vi "resampleA.vi"(8 "error in (no error)":errorcluster, 11 "Waveform":waveform(dbl)) -> (0 "error out":errorcluster, 3 "resampled waveform out":waveform(dbl))   [LabVIEW 2018]
uses:
  <vilib>/measure/maresamp.llb/Resample Waveform (single shot).vi
  <vilib>/measure/NI_MAPro.lvlib
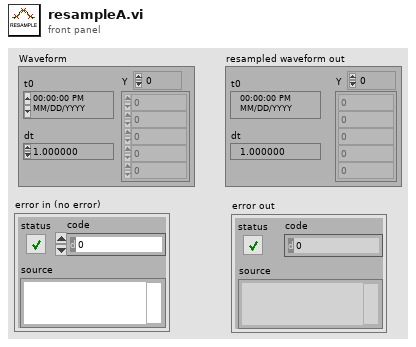
[diagram p1: front panel]
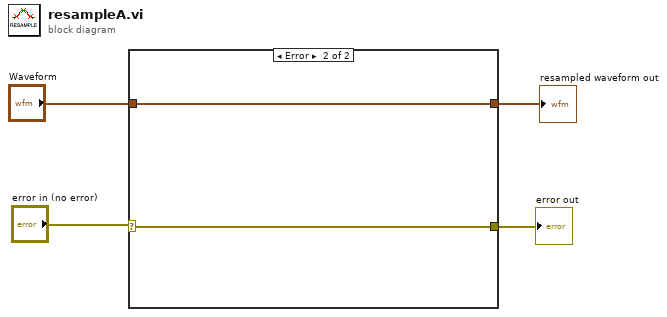
[diagram p0: block diagram]
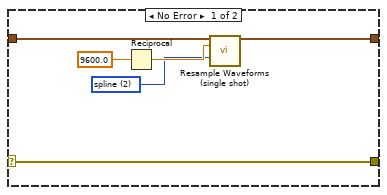
[diagram p2: hidden frame]
diagram:
  n1 = case shown="Error" "error in (no error)" {
    selector: "error in (no error)" -> [w5 w12]
    tunnel: [w10 w11] -> w4
    tunnel: "Waveform" -> [w6 w11]
    tunnel: [w5 w12] -> w1
    frame No Error {
      w7 = u16 2 items=["coerce", "linear", "spline", "FIR filter"] ("interpolation mode")
      n2 = Reciprocal(x=9600.0) -> (1/x=w9:dbl)
      n3 = call-poly <vilib>:"Resample Waveforms (single shot).vi"("waveform in"=w6, "dt"=w9, "interpolation mode"=w7) -> ("resampled waveform out"=w10:waveform(dbl))  [unwired: 9 in, 3 out]
    }
    frame Error {
    }
  }
  "resampled waveform out" <- w4
  "error out" <- w1
